vi "LM 3D Gaussian ACF and gradient.vi"(3 "output control":T1, 4 "data":variant, 5 "X":dbl[](array[numeric]), 6 "a":dbl[](array[numeric])) -> (0 "error out":errorcluster, 1 "f'(X,a)":dbl[][](array[numeric]), 2 "f(X,a)":dbl[](array[numeric]))   [LabVIEW 2021, in "Fits.lvlib"]
doc: "This template is the starting point for creating a model function to be passed to the Nonlinear Curve Fit.vi."
uses:
  <vilib>/gmath/NumericalOptimization/LM_output select.ctl
  Fits.lvlib
  <vilib>/gmath/NI_Gmath.lvlib
panel:
  # "Parameters:\n\namplitude: A\ndiffusion time: t\naspect ratio: w"
  # "f(x) = 1 + A/(1+x/t)/(1+x/w^2*t)^1/2"
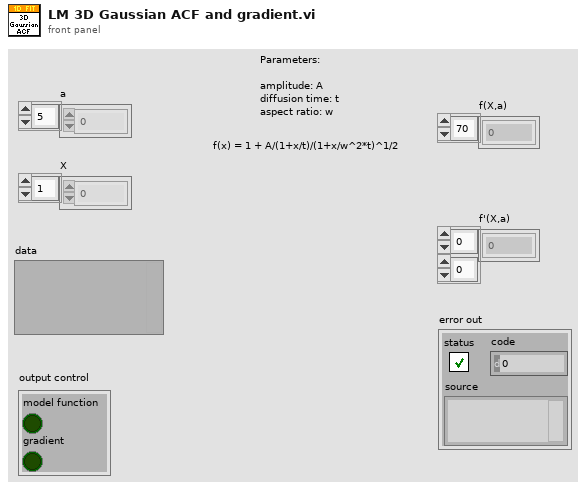
[diagram p1: front panel]
types:
  T1 = typedef "NI_Gmath.lvlib/LM_output select.ctl" = cluster{"model function":bool, "gradient":bool}
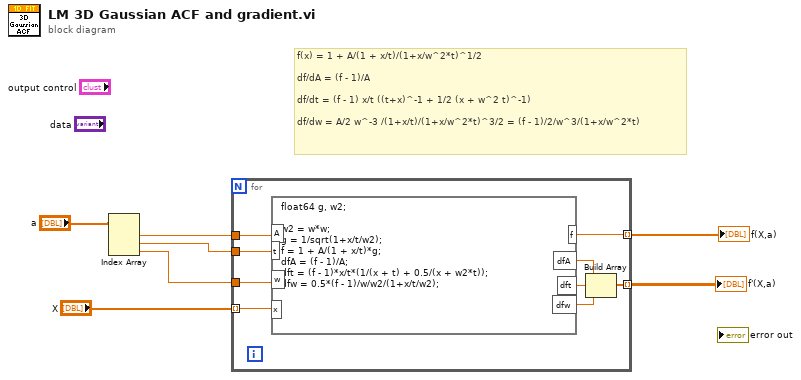
[diagram p0: block diagram]
diagram:
  # "f(x) = 1 + A/(1 + x/t)/(1+x/w^2*t)^1/2\n\ndf/dA = (f - 1)/A\n\ndf/dt = (f - 1) x/t ((t+x)^-1 + 1/2 (x + w^2 t)^-1)\n\ndf/dw = A/2 w^-3 /(1+x/t)/(1+x/w^2*t)^3/2 = (f - 1)/2/w^3/(1+x/w^2*t)"
  n1 = Index Array(array="a") -> (element #1=w3:dbl, element #2=w2:dbl, element #3=w1:dbl)  [unwired: 3 in]
  n2 = for {
    tunnel: w3 -> [w15]
    tunnel: w2 -> [w16]
    tunnel: "X" -> [w14] mode=indexing
    tunnel: [w13] -> w5 mode=indexing
    tunnel: [w10] -> w4 mode=indexing
    tunnel: w1 -> [w9]
    n3 = formula code="float64 g, w2;\n\nw2 = w*w;\ng = 1/sqrt(1+x/t/w2);\nf = 1 + A/(1 + x/t)*g;\ndfA = (f - 1)/A;\ndft = (f - 1)*x/t*(1/(x + t) + 0.5/(x + w2*t));\ndfw = 0.5*(f - 1)/w/w2/(1+x/t/w2);"("A"=w15, "t"=w16, "x"=w14, "w"=w9) -> ("f"=w13:dbl, "dfA"=w12:dbl, "dft"=w11:dbl, "dfw"=w8:dbl)
    n4 = Build Array(w12, w11, w8) -> (w10:dbl[])
  }
  "f(X,a)" <- w5
  "f'(X,a)" <- w4
